vi "Remove All Endpoint Configurations.vi"(8 "error in":errorcluster, 11 "endpoint configuration in":T1 format="%.0x") -> (0 "error out":errorcluster, 3 "endpoint configuration out":T1 format="%.0x")   [LabVIEW 2020, in "SLSC Switch Scripting.lvlib"]
uses:
  SLSC Switch Scripting.lvlib
  <vilib>/NI VeriStand/Custom Device API/Custom Device Item Ref.ctl
  <vilib>/NI VeriStand/Custom Device API/Custom Device API.lvlib
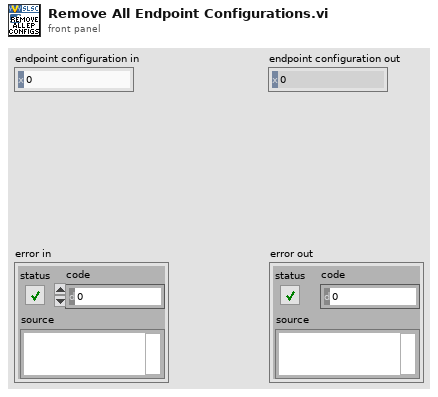
[diagram p1: front panel]
types:
  T1 = typedef "Custom Device API.lvlib/Custom Device Item Ref.ctl" = u64
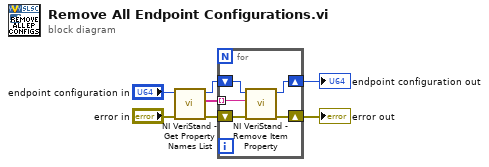
[diagram p0: block diagram]
diagram:
  n1 = call <vilib>:"NI VeriStand - Get Property Names List.vi"("error in (no error)"="error in", "Item Ref in"="endpoint configuration in") -> ("error out"=w5:errorcluster, "Property Names"=w3:string[], "Item Ref out"=w2:T1)  [unwired: 7 in]
  n2 = for {
    tunnel: w3 -> [w10] mode=indexing
    shift-right: [w11] -> w4
    shift-left: w5 -> [w12]
    shift-right: [w8] -> w1
    shift-left: w2 -> [w9]
    n3 = call <vilib>:"NI VeriStand - Remove Item Property.vi"("error in (no error)"=w12, "Property Name"=w10, "Item Ref in"=w9) -> ("error out"=w11:errorcluster, "Item Ref out"=w8:T1)  [unwired: 6 in, 1 out]
  }
  "error out" <- w4
  "endpoint configuration out" <- w1
